vi "FPGA Top Level.vi"() -> ()   [LabVIEW 2016]
doc: "A LabVIEW implementation of <b>FPGA4Fun</b>'s Music Box series."
uses:
  <vilib>/Platform/TimedLoop/XDataNode/timing_clust.ctl
  <vilib>/Platform/TimedLoop/XDataNode/nitl_modes.ctl
  <vilib>/Platform/TimedLoop/XDataNode/wakeup.ctl
  <vilib>/rvi/Emulation/niFpgaGetClockAttributes.vi
  <vilib>/rvi/Emulation/niFpgaSctlEmulationGetInTimedLoop.vi
  <vilib>/rvi/Emulation/niFpgaEmulationReportErrorSimple.vi
  <vilib>/rvi/eio/common/nirviEmuTemplateMethod_errors.vi
  <vilib>/rvi/Emulation/niFpgaCriticalErrorInLSC.vi
  <vilib>/rvi/Emulation/niFpgaProcessEmulError.vi
  <vilib>/eio/EIONode/EIONode.xnode
  <vilib>/Platform/TimedLoop/XDataNode/XDataNode.xnode
  <vilib>/Platform/TimedLoop/XDataNode/XDNodeRunTimeDep.lvlib
panel:
  in  "Array":bool[](array[boolean])=[FALSE, FALSE, FALSE, FALSE, FALSE, FALSE, FALSE, FALSE, FALSE, FALSE, FALSE, FALSE]
  out "Boolean array\nas number":u32 format="%b"
  out "Boolean array":bool[](array[boolean])
  out "C":bool
  out "B":bool
  out "Bb":bool
  out "A":bool
  out "Ab":bool
  out "G":bool
  out "Gb":bool
  out "F":bool
  out "E":bool
  out "Eb":bool
  out "D":bool
  out "Db":bool
  in  "Volume":i16(knob)=2 scale=0.0..100.0
  # "Warning: Careful when using headphones, this example can be very loud!"
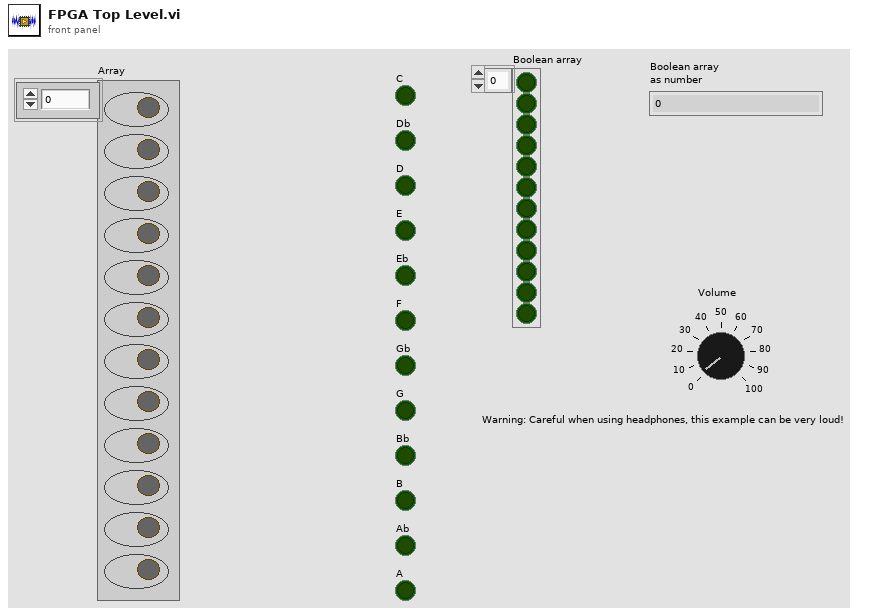
[diagram p1: front panel]
types:
  T1 = typedef "XDNodeRunTimeDep.lvlib/timing_clust.ctl" = cluster{"Expected End [f-1]":u64, "Actual End [f-1]":u64, "Finished Late? [f-1]":bool, "Expected End [i-1]":u64, "Actual End [i-1]":u64, "Finished Late? [i-1]":bool, "Expected Start [i]":u64, "Actual Start [i]":u64, "Expected Start [f]":u64, "Actual Start [f]":u64, "Source Name":string, "Structure Name":string, "Period":i64, "Deadline":i64, "Offset":i64, "Start":i64, "Priority":i32, "Timeout":i32, "Mode":T2, "Wakeup Reason":T3, "Error":errorcluster, "Source Type":string, "Secondary Source Type":string, "Global End Time":u64, "Global Start Time":u64, "Frame Duration":u64, "Iteration Duration":u64, "Assigned CPU":i32, "I/O Scan Engine Mode":u32}
  T2 = typedef "XDNodeRunTimeDep.lvlib/nitl_modes.ctl" = enum32{"No Change", "Process missed periods, maintain original phase", "Discard missed periods, maintain original phase", "Process missed periods, ignore original phase", "Discard missed periods, ignore original phase"}
  T3 = typedef "XDNodeRunTimeDep.lvlib/wakeup.ctl" = enum32{"Normal", "Aborted", "Asynchronous wakeup", "Timing source error", "Timed loop error", "Timeout"}
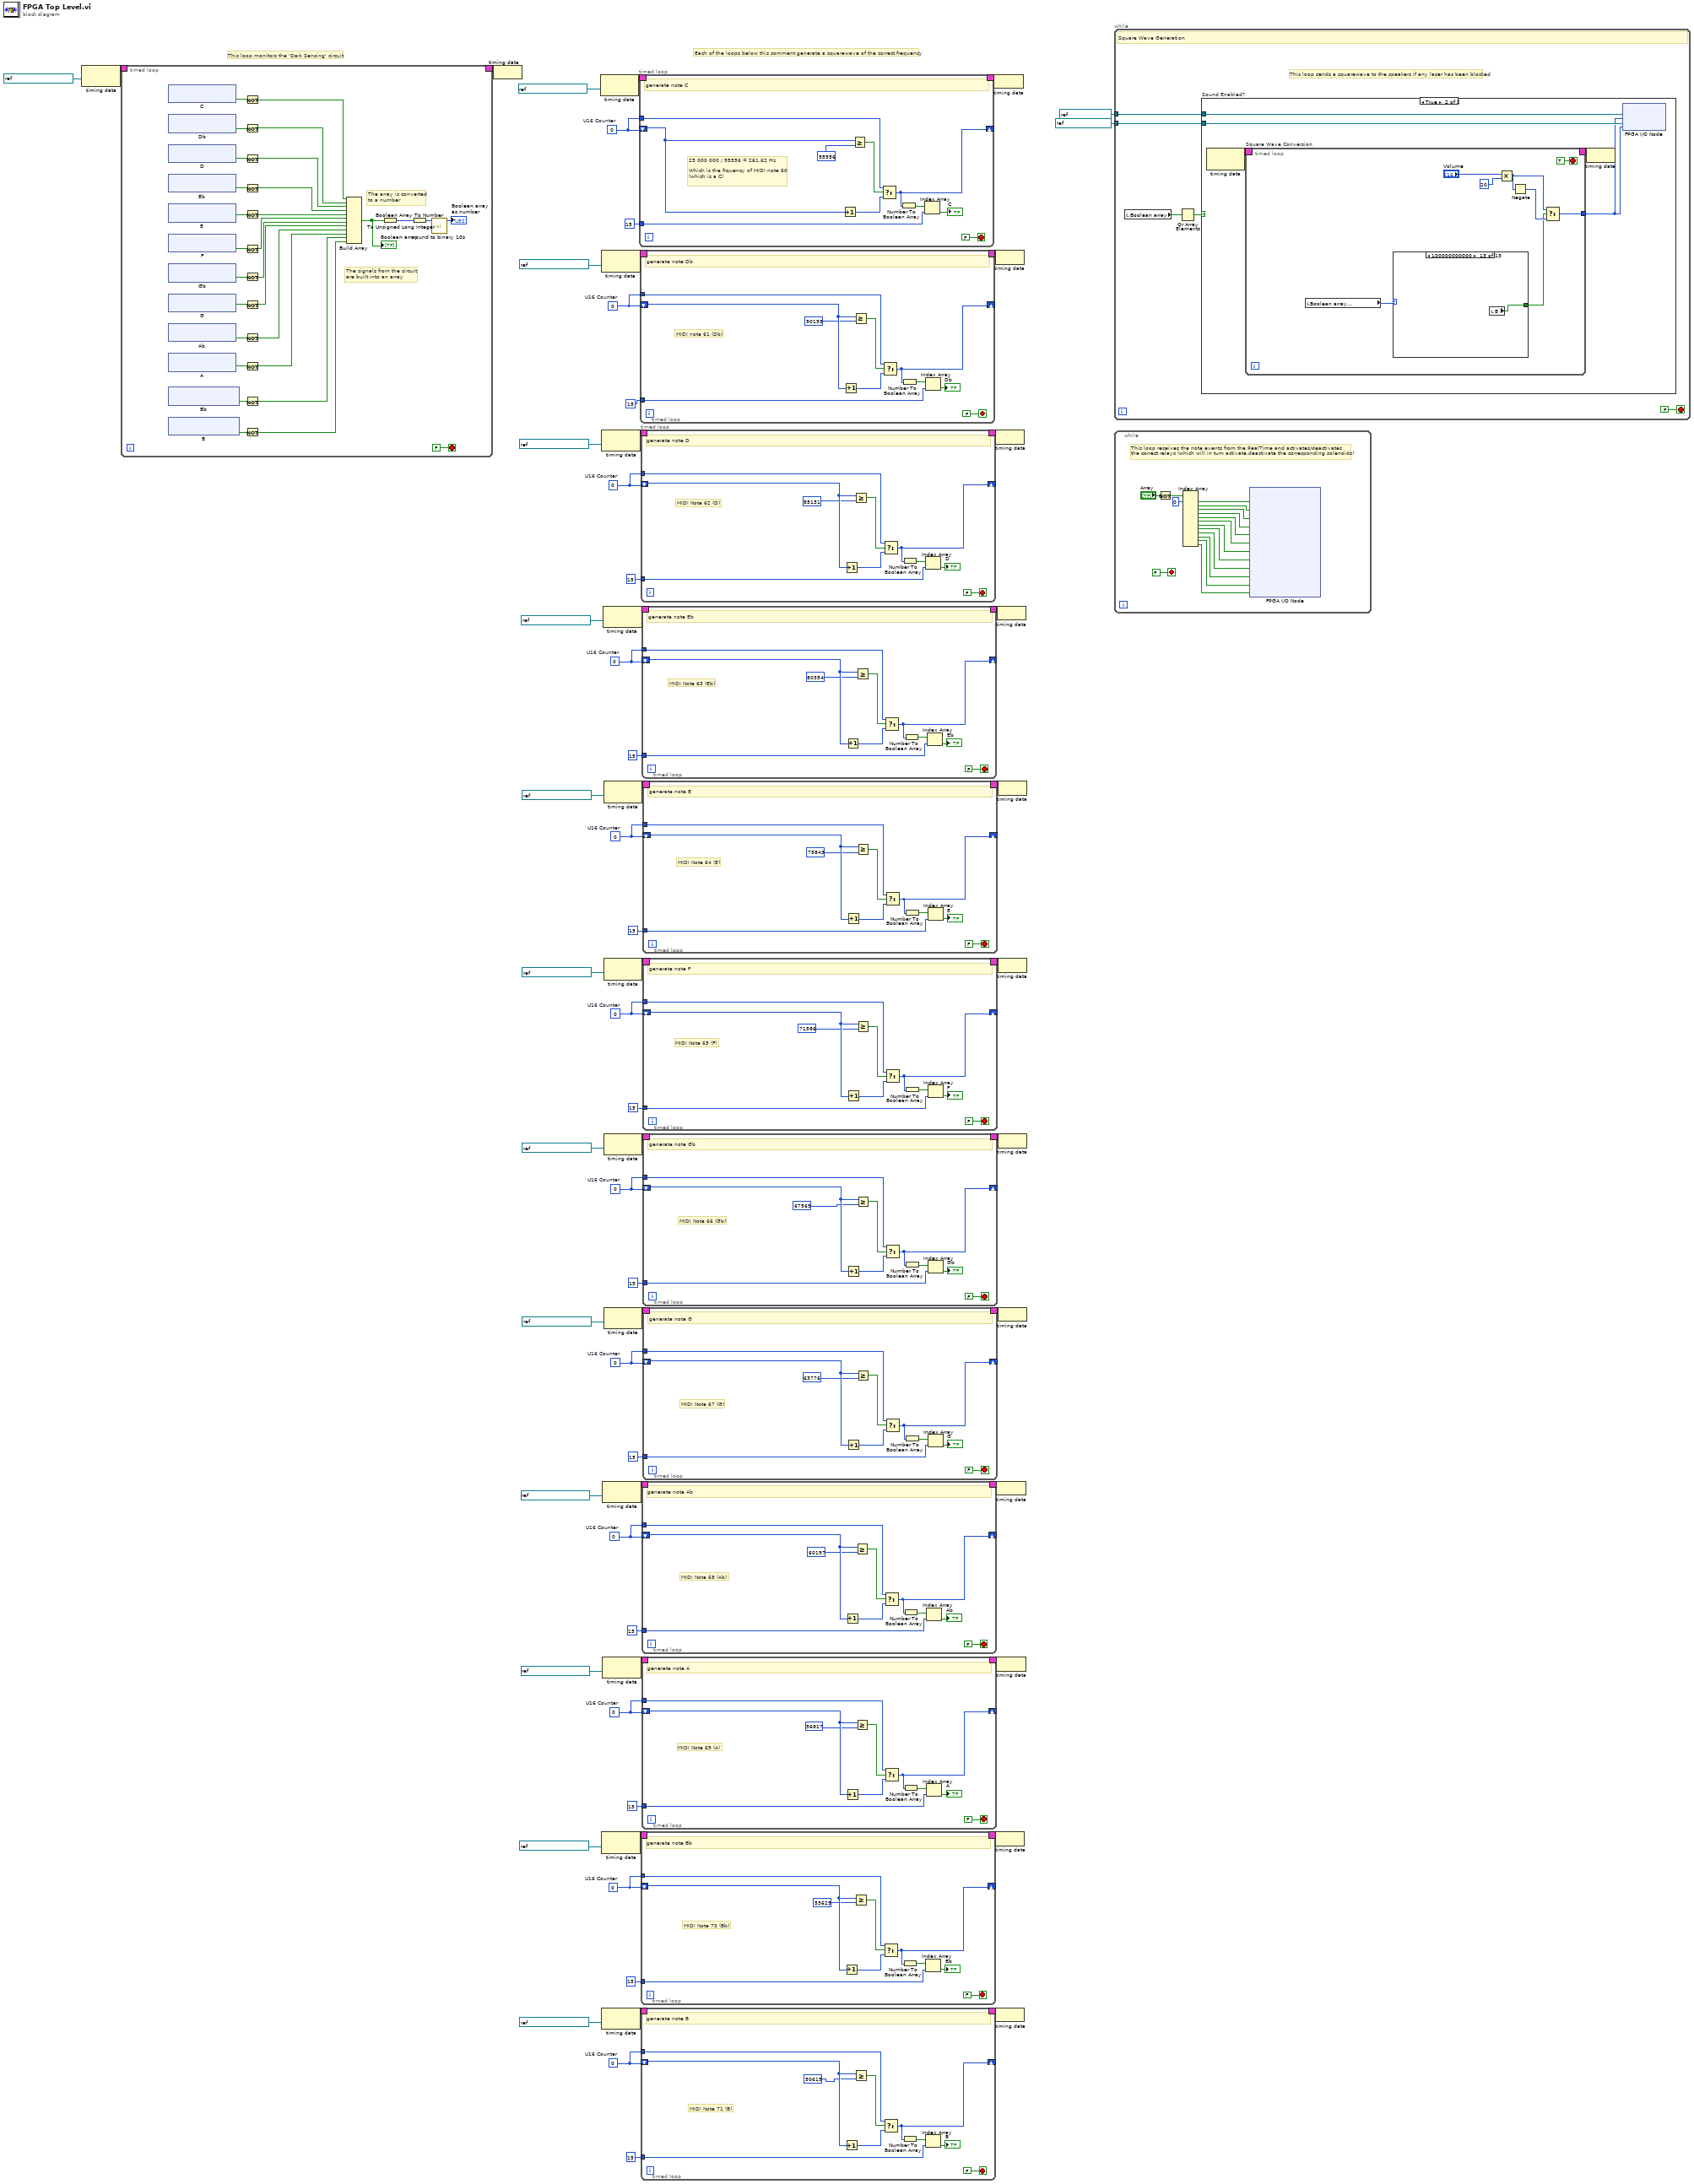
[diagram p0: block diagram]
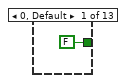
[diagram p3: hidden frame]
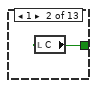
[diagram p4: hidden frame]
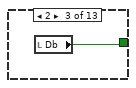
[diagram p5: hidden frame]
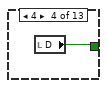
[diagram p6: hidden frame]
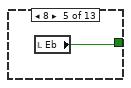
[diagram p7: hidden frame]
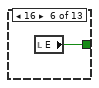
[diagram p8: hidden frame]
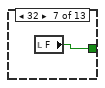
[diagram p9: hidden frame]
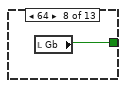
[diagram p10: hidden frame]
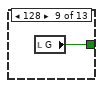
[diagram p11: hidden frame]
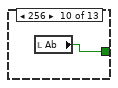
[diagram p12: hidden frame]
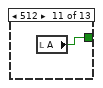
[diagram p13: hidden frame]
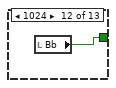
[diagram p14: hidden frame]
diagram:
  w6 = u32 0  # U16 Counter
  w11 = u32 0  # U16 Counter
  w16 = u32 0  # U16 Counter
  w21 = u32 0  # U16 Counter
  w26 = u32 0  # U16 Counter
  w31 = u32 0  # U16 Counter
  w36 = u32 0  # U16 Counter
  w41 = u32 0  # U16 Counter
  w46 = u32 0  # U16 Counter
  w49 = u32 0  # U16 Counter
  w56 = u32 0  # U16 Counter
  w61 = u32 0  # U16 Counter
  # "Each of the loops below this comment generate a squarewave of the correct frequency"
  # "This loop monitors the 'Dark Sensing' circuit"
  n1 = node-c288(refnum<k21> "25MHz Derived Clock" ("Source Name")) -> (w3:T1)
  n2 = timed-loop {
    timing: w3 -> [_]
    timing-out: [_] -> w2
    stop <- FALSE stop-if-true
    # "The array is converted\nto a number"
    # "The signals from the circuit\nare built into an array"
    n3 = xnode "C"() -> ("ConnectorB/DIO0"=w94:bool)  [unwired: 1 in, 1 out]
    n4 = xnode "Db"() -> ("ConnectorB/DIO1"=w93:bool)  [unwired: 1 in, 1 out]
    n5 = xnode "D"() -> ("ConnectorB/DIO2"=w85:bool)  [unwired: 1 in, 1 out]
    n6 = xnode "Eb"() -> ("ConnectorB/DIO3"=w92:bool)  [unwired: 1 in, 1 out]
    n7 = xnode "E"() -> ("ConnectorB/DIO4"=w91:bool)  [unwired: 1 in, 1 out]
    n8 = xnode "F"() -> ("ConnectorB/DIO5"=w86:bool)  [unwired: 1 in, 1 out]
    n9 = xnode "Gb"() -> ("ConnectorB/DIO6"=w90:bool)  [unwired: 1 in, 1 out]
    n10 = xnode "G"() -> ("ConnectorB/DIO7"=w89:bool)  [unwired: 1 in, 1 out]
    n11 = xnode "Ab"() -> ("ConnectorB/DIO8"=w84:bool)  [unwired: 1 in, 1 out]
    n12 = xnode "A"() -> ("ConnectorB/DIO9"=w88:bool)  [unwired: 1 in, 1 out]
    n13 = xnode "Bb"() -> ("ConnectorB/DIO10"=w87:bool)  [unwired: 1 in, 1 out]
    n14 = xnode "B"() -> ("ConnectorB/DIO11"=w83:bool)  [unwired: 1 in, 1 out]
    n15 = Not(x=w94) -> (.not. x?=w80:bool)
    n16 = Not(x=w93) -> (.not. x?=w79:bool)
    n17 = Not(x=w85) -> (.not. x?=w78:bool)
    n18 = Not(x=w92) -> (.not. x?=w77:bool)
    n19 = Not(x=w91) -> (.not. x?=w76:bool)
    n20 = Not(x=w86) -> (.not. x?=w75:bool)
    n21 = Not(x=w90) -> (.not. x?=w74:bool)
    n22 = Not(x=w89) -> (.not. x?=w73:bool)
    n23 = Not(x=w84) -> (.not. x?=w72:bool)
    n24 = Not(x=w88) -> (.not. x?=w71:bool)
    n25 = Not(x=w87) -> (.not. x?=w70:bool)
    n26 = Not(x=w83) -> (.not. x?=w69:bool)
    n27 = Build Array(w80, w79, w78, w77, w76, w75, w74, w73, w72, w71, w70, w69) -> (w81:bool[])
    "Boolean array" <- w81
    n28 = Boolean Array To Number(Boolean array=w81) -> (number=w68:u16)
    n29 = To Unsigned Long Integer(number=w68) -> (unsigned 32bit integer=w67:u32)
    n30 = call "round to binary 10s.vi"("Numeric"=w67) -> ("Numeric 2"=→"Boolean array\nas number":u32)  [unwired: 10 in]
  }
  n31 = node-c288(w2) -> ()
  n32 = node-c288(refnum<k21> "25MHz Derived Clock" ("Source Name")) -> (w65:T1)
  n33 = node-c288(refnum<k21> "25MHz Derived Clock" ("Source Name")) -> (w58:T1)
  n34 = node-c288(refnum<k21> "25MHz Derived Clock" ("Source Name")) -> (w53:T1)
  n35 = node-c288(refnum<k21> "25MHz Derived Clock" ("Source Name")) -> (w13:T1)
  n36 = node-c288(refnum<k21> "25MHz Derived Clock" ("Source Name")) -> (w8:T1)
  n37 = node-c288(refnum<k21> "25MHz Derived Clock" ("Source Name")) -> (w23:T1)
  n38 = node-c288(refnum<k21> "25MHz Derived Clock" ("Source Name")) -> (w18:T1)
  n39 = node-c288(refnum<k21> "25MHz Derived Clock" ("Source Name")) -> (w48:T1)
  n40 = node-c288(refnum<k21> "25MHz Derived Clock" ("Source Name")) -> (w43:T1)
  n41 = node-c288(refnum<k21> "25MHz Derived Clock" ("Source Name")) -> (w38:T1)
  n42 = node-c288(refnum<k21> "25MHz Derived Clock" ("Source Name")) -> (w33:T1)
  n43 = node-c288(refnum<k21> "25MHz Derived Clock" ("Source Name")) -> (w28:T1)
  n44 = timed-loop {
    timing: w65 -> [_]
    timing-out: [_] -> w64
    shift-right: [w102] -> _
    shift-left: w61 -> [w99]
    tunnel: 15 -> [w101]
    tunnel: w61 -> [w100]
    stop <- FALSE stop-if-true
    # "25 000 000 / 95556 = 261.62 Hz\n\nWhich is the frquency of MIDI note 60\n(which is a C)"
    # "generate note C"
    n45 = Increment(x=w99) -> (x+1=w104:u32)
    n46 = Greater Or Equal?(x=w99, y=u32 95556) -> (x >= y?=w105:bool)
    n47 = Select(t=w100, s=w105, f=w104) -> (s? t:f=w102:u32)
    n48 = Number To Boolean Array(number=w102) -> (Boolean array=w103:bool[])
    n49 = Index Array(array=w103, index=w101) -> (element=→"C":bool)
  }
  n50 = timed-loop {
    timing: w58 -> [_]
    timing-out: [_] -> w57
    shift-right: [w114] -> _
    shift-left: w56 -> [w110]
    tunnel: 15 -> [w113]
    tunnel: w56 -> [w112]
    stop <- FALSE stop-if-true
    # "MIDI note 61 (Db)"
    # "generate note Db"
    n51 = Increment(x=w110) -> (x+1=w116:u32)
    n52 = Greater Or Equal?(x=w110, y=u32 90193) -> (x >= y?=w117:bool)
    n53 = Select(t=w112, s=w117, f=w116) -> (s? t:f=w114:u32)
    n54 = Number To Boolean Array(number=w114) -> (Boolean array=w115:bool[])
    n55 = Index Array(array=w115, index=w113) -> (element=→"Db":bool)
  }
  n56 = timed-loop {
    timing: w53 -> [_]
    timing-out: [_] -> w52
    shift-right: [w126] -> _
    shift-left: w49 -> [w122]
    tunnel: 15 -> [w125]
    tunnel: w49 -> [w124]
    stop <- FALSE stop-if-true
    # "MIDI Note 62 (D)"
    # "generate note D"
    n57 = Increment(x=w122) -> (x+1=w128:u32)
    n58 = Greater Or Equal?(x=w122, y=u32 85131) -> (x >= y?=w129:bool)
    n59 = Select(t=w124, s=w129, f=w128) -> (s? t:f=w126:u32)
    n60 = Number To Boolean Array(number=w126) -> (Boolean array=w127:bool[])
    n61 = Index Array(array=w127, index=w125) -> (element=→"D":bool)
  }
  n62 = timed-loop {
    timing: w13 -> [_]
    timing-out: [_] -> w12
    shift-right: [w138] -> _
    shift-left: w11 -> [w134]
    tunnel: 15 -> [w137]
    tunnel: w11 -> [w136]
    stop <- FALSE stop-if-true
    # "MIDI Note 70 (Bb)"
    # "generate note Bb"
    n63 = Increment(x=w134) -> (x+1=w140:u32)
    n64 = Greater Or Equal?(x=w134, y=u32 53629) -> (x >= y?=w141:bool)
    n65 = Select(t=w136, s=w141, f=w140) -> (s? t:f=w138:u32)
    n66 = Number To Boolean Array(number=w138) -> (Boolean array=w139:bool[])
    n67 = Index Array(array=w139, index=w137) -> (element=→"Bb":bool)
  }
  n68 = timed-loop {
    timing: w8 -> [_]
    timing-out: [_] -> w7
    shift-right: [w150] -> _
    shift-left: w6 -> [w146]
    tunnel: 15 -> [w149]
    tunnel: w6 -> [w148]
    stop <- FALSE stop-if-true
    # "MIDI Note 71 (B)"
    # "generate note B"
    n69 = Increment(x=w146) -> (x+1=w152:u32)
    n70 = Greater Or Equal?(x=w146, y=u32 50619) -> (x >= y?=w153:bool)
    n71 = Select(t=w148, s=w153, f=w152) -> (s? t:f=w150:u32)
    n72 = Number To Boolean Array(number=w150) -> (Boolean array=w151:bool[])
    n73 = Index Array(array=w151, index=w149) -> (element=→"B":bool)
  }
  n74 = timed-loop {
    timing: w23 -> [_]
    timing-out: [_] -> w22
    shift-right: [w162] -> _
    shift-left: w21 -> [w158]
    tunnel: 15 -> [w161]
    tunnel: w21 -> [w160]
    stop <- FALSE stop-if-true
    # "MIDI Note 68 (Ab)"
    # "generate note Ab"
    n75 = Increment(x=w158) -> (x+1=w164:u32)
    n76 = Greater Or Equal?(x=w158, y=u32 60197) -> (x >= y?=w165:bool)
    n77 = Select(t=w160, s=w165, f=w164) -> (s? t:f=w162:u32)
    n78 = Number To Boolean Array(number=w162) -> (Boolean array=w163:bool[])
    n79 = Index Array(array=w163, index=w161) -> (element=→"Ab":bool)
  }
  n80 = timed-loop {
    timing: w18 -> [_]
    timing-out: [_] -> w17
    shift-right: [w174] -> _
    shift-left: w16 -> [w170]
    tunnel: 15 -> [w173]
    tunnel: w16 -> [w172]
    stop <- FALSE stop-if-true
    # "MIDI Note 69 (A)"
    # "generate note A"
    n81 = Increment(x=w170) -> (x+1=w176:u32)
    n82 = Greater Or Equal?(x=w170, y=u32 56817) -> (x >= y?=w177:bool)
    n83 = Select(t=w172, s=w177, f=w176) -> (s? t:f=w174:u32)
    n84 = Number To Boolean Array(number=w174) -> (Boolean array=w175:bool[])
    n85 = Index Array(array=w175, index=w173) -> (element=→"A":bool)
  }
  n86 = timed-loop {
    timing: w48 -> [_]
    timing-out: [_] -> w47
    shift-right: [w186] -> _
    shift-left: w46 -> [w182]
    tunnel: 15 -> [w185]
    tunnel: w46 -> [w184]
    stop <- FALSE stop-if-true
    # "MIDI Note 63 (Eb)"
    # "generate note Eb"
    n87 = Increment(x=w182) -> (x+1=w188:u32)
    n88 = Greater Or Equal?(x=w182, y=u32 80354) -> (x >= y?=w189:bool)
    n89 = Select(t=w184, s=w189, f=w188) -> (s? t:f=w186:u32)
    n90 = Number To Boolean Array(number=w186) -> (Boolean array=w187:bool[])
    n91 = Index Array(array=w187, index=w185) -> (element=→"Eb":bool)
  }
  n92 = timed-loop {
    timing: w43 -> [_]
    timing-out: [_] -> w42
    shift-right: [w198] -> _
    shift-left: w41 -> [w194]
    tunnel: 15 -> [w197]
    tunnel: w41 -> [w196]
    stop <- FALSE stop-if-true
    # "MIDI Note 64 (E)"
    # "generate note E"
    n93 = Increment(x=w194) -> (x+1=w200:u32)
    n94 = Greater Or Equal?(x=w194, y=u32 75843) -> (x >= y?=w201:bool)
    n95 = Select(t=w196, s=w201, f=w200) -> (s? t:f=w198:u32)
    n96 = Number To Boolean Array(number=w198) -> (Boolean array=w199:bool[])
    n97 = Index Array(array=w199, index=w197) -> (element=→"E":bool)
  }
  n98 = timed-loop {
    timing: w38 -> [_]
    timing-out: [_] -> w37
    shift-right: [w210] -> _
    shift-left: w36 -> [w206]
    tunnel: 15 -> [w209]
    tunnel: w36 -> [w208]
    stop <- FALSE stop-if-true
    # "MIDI Note 65 (F)"
    # "generate note F"
    n99 = Increment(x=w206) -> (x+1=w212:u32)
    n100 = Greater Or Equal?(x=w206, y=u32 71586) -> (x >= y?=w213:bool)
    n101 = Select(t=w208, s=w213, f=w212) -> (s? t:f=w210:u32)
    n102 = Number To Boolean Array(number=w210) -> (Boolean array=w211:bool[])
    n103 = Index Array(array=w211, index=w209) -> (element=→"F":bool)
  }
  n104 = timed-loop {
    timing: w33 -> [_]
    timing-out: [_] -> w32
    shift-right: [w222] -> _
    shift-left: w31 -> [w218]
    tunnel: 15 -> [w221]
    tunnel: w31 -> [w220]
    stop <- FALSE stop-if-true
    # "MIDI Note 66 (Gb)"
    # "generate note Gb"
    n105 = Increment(x=w218) -> (x+1=w224:u32)
    n106 = Greater Or Equal?(x=w218, y=u32 67569) -> (x >= y?=w225:bool)
    n107 = Select(t=w220, s=w225, f=w224) -> (s? t:f=w222:u32)
    n108 = Number To Boolean Array(number=w222) -> (Boolean array=w223:bool[])
    n109 = Index Array(array=w223, index=w221) -> (element=→"Gb":bool)
  }
  n110 = timed-loop {
    timing: w28 -> [_]
    timing-out: [_] -> w27
    shift-right: [w234] -> _
    shift-left: w26 -> [w230]
    tunnel: 15 -> [w233]
    tunnel: w26 -> [w232]
    stop <- FALSE stop-if-true
    # "MIDI Note 67 (G)"
    # "generate note G"
    n111 = Increment(x=w230) -> (x+1=w236:u32)
    n112 = Greater Or Equal?(x=w230, y=u32 63776) -> (x >= y?=w237:bool)
    n113 = Select(t=w232, s=w237, f=w236) -> (s? t:f=w234:u32)
    n114 = Number To Boolean Array(number=w234) -> (Boolean array=w235:bool[])
    n115 = Index Array(array=w235, index=w233) -> (element=→"G":bool)
  }
  n116 = node-c288(w64) -> ()
  n117 = node-c288(w57) -> ()
  n118 = node-c288(w52) -> ()
  n119 = node-c288(w12) -> ()
  n120 = node-c288(w7) -> ()
  n121 = node-c288(w22) -> ()
  n122 = node-c288(w17) -> ()
  n123 = node-c288(w47) -> ()
  n124 = node-c288(w42) -> ()
  n125 = node-c288(w37) -> ()
  n126 = node-c288(w32) -> ()
  n127 = node-c288(w27) -> ()
  n128 = while {
    tunnel: refnum<k21> "AudioOut/Left" ("FPGA I/O In") -> [w243]
    tunnel: refnum<k21> "AudioOut/Right" ("FPGA I/O In") -> [w244]
    stop <- FALSE stop-if-true
    # "This loop sends a squarewave to the speakers if any laser has been blocked"
    # "Square Wave Generation"
    n129 = local read "Boolean array"() -> (w242:bool[])
    n130 = Or Array Elements(Boolean array=w242) -> (logical OR=w241:bool)
    n131 = case "Sound Enabled?" shown="True" w241 {
      tunnel: w244 -> [_ w250]
      tunnel: w243 -> [_ w249]
      frame False {
      }
      frame True {
        n132 = node-c288() -> (w247:T1)  [unwired: 1 in]
        n133 = timed-loop "Square Wave Conversion" {
          timing: w247 -> [_]
          timing-out: [_] -> w246
          tunnel: [w254] -> w248
          stop <- TRUE stop-if-true
          n134 = local read "Boolean array\nas number"() -> (w251:u32)
          n135 = case shown="100000000000" w251 {
            tunnel: [FALSE ("C") w260 w261 w262 w263 w264 w265 w266 w267 w268 w269 w270 w271] -> w252
            frame 0, Default {
            }
            frame 1 {
              n136 = local read "C"() -> (w260:bool)
            }
            frame 2 {
              n137 = local read "Db"() -> (w261:bool)
            }
            frame 4 {
              n138 = local read "D"() -> (w262:bool)
            }
            frame 8 {
              n139 = local read "Eb"() -> (w263:bool)
            }
            frame 16 {
              n140 = local read "E"() -> (w264:bool)
            }
            frame 32 {
              n141 = local read "F"() -> (w265:bool)
            }
            frame 64 {
              n142 = local read "Gb"() -> (w266:bool)
            }
            frame 128 {
              n143 = local read "G"() -> (w267:bool)
            }
            frame 256 {
              n144 = local read "Ab"() -> (w268:bool)
            }
            frame 512 {
              n145 = local read "A"() -> (w269:bool)
            }
            frame 1024 {
              n146 = local read "Bb"() -> (w270:bool)
            }
            frame 2048 {
              n147 = local read "B"() -> (w271:bool)
            }
          }
          n148 = Multiply(x="Volume", y=i16 20 ("Volume 2")) -> (x*y=w256:i16)
          n149 = Negate(x=w256) -> (-x=w255:i16)
          n150 = Select(t=w256, s=w252, f=w255) -> (s? t:f=w254:i16)
        }
        n151 = node-c288(w246) -> ()
        n152 = xnode "FPGA I/O Node"("I/O Item"=w248, "FPGA I/O In"=w249, "I/O Item"=w248, "FPGA I/O In"=w250) -> ()  [unwired: 2 out]
      }
    }
  }
  n153 = while {
    stop <- FALSE stop-if-true
    # "This loop receives the note events from the RealTime and activates/deactivates\nthe correct relays (which will in turn activate.deactivate the corresponding solenoids)"
    n154 = Not(x="Array") -> (.not. x?=w289:bool[])
    n155 = Index Array(array=w289, index #1=0 ("index")) -> (element #1=w287:bool, element #2=w286:bool, element #3=w285:bool, element #4=w284:bool, element #5=w283:bool, element #6=w282:bool, element #7=w281:bool, element #8=w280:bool, element #9=w279:bool, element #10=w278:bool, element #11=w277:bool, element #12=w276:bool)  [unwired: 11 in]
    n156 = xnode "FPGA I/O Node"("ConnectorA/DIO0"=w287, "ConnectorA/DIO1"=w286, "ConnectorA/DIO2"=w285, "ConnectorA/DIO3"=w284, "ConnectorA/DIO4"=w283, "ConnectorA/DIO5"=w282, "ConnectorA/DIO6"=w281, "ConnectorA/DIO7"=w280, "ConnectorA/DIO8"=w279, "ConnectorA/DIO9"=w278, "ConnectorA/DIO10"=w277, "ConnectorA/DIO15"=w276) -> ()  [unwired: 12 in, 12 out]
  }
